vi "MDrive_Get_Variable.vi"(3 "error in":errorcluster, 4 "Variable":string, 5 "VISA resource name in":refnum<visa-resource-name>) -> (0 "error out":errorcluster, 1 "number":i32, 2 "VISA resource name out":refnum<visa-resource-name>)   [LabVIEW 2010]
panel:
  out "substring":string
  out "String":string="\r\n"
  out "return count":u32
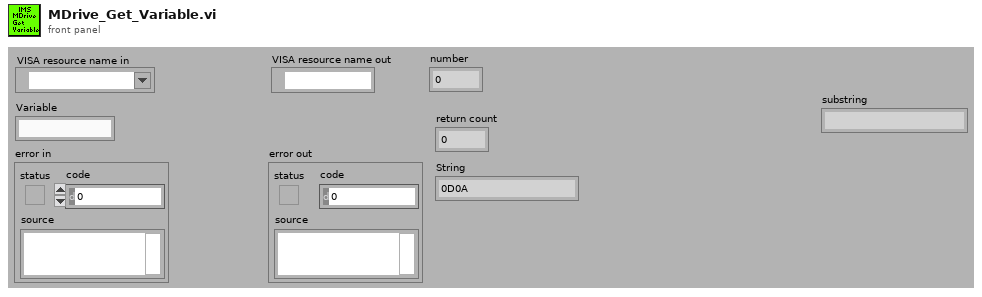
[diagram p1: front panel]
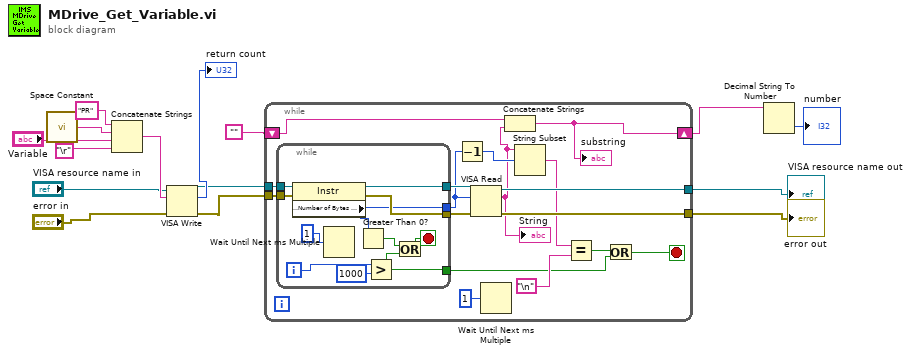
[diagram p0: block diagram]
diagram:
  n1 = call <vilib>:"Space Constant.vi"() -> ("String"=w12:string)
  n2 = Concatenate Strings("PR" ("string"), w12, "Variable", "\r") -> (w15:string)
  n3 = VISA Write(VISA resource name="VISA resource name in", write buffer=w15, error in (no error)="error in") -> (VISA resource name out=w6:refnum<visa-resource-name>, return count=→"return count":u32, error out=w5:errorcluster)
  n4 = while {
    tunnel: w6 -> [w30]
    tunnel: w5 -> [w29]
    tunnel: [w28] -> w3
    tunnel: [w27] -> w2
    shift-right: [w21] -> w1
    shift-left: "" -> [w22]
    stop <- w17 stop-if-true
    n5 = while {
      tunnel: [w43] -> w32
      tunnel: [w42] -> w31
      tunnel: w30 -> [w41]
      tunnel: w29 -> [w40]
      tunnel: [w39] -> w25
      tunnel: [w33] -> w18
      i -> [w37]
      stop <- w34 stop-if-true
      n6 = property class="Instr"(reference=w41, error in=w40) -> (reference out=w43:refnum<visa-resource-name>, error out=w42:errorcluster, "Serial Settings:Number of Bytes at Serial Port"=w39:u32)
      n7 = Wait Until Next ms Multiple(millisecond multiple=u32 1) -> ()  [unwired: 1 out]
      n8 = Greater Than 0?(x=w39) -> (x > 0?=w35:bool)
      n9 = Greater?(x=w37, y=1000) -> (0:w33:bool)
      n10 = Or(x=w35, y=w33) -> (x .or. y?=w34:bool)
    }
    n11 = Decrement(x=w25) -> (x-1=w24:u32)
    n12 = VISA Read(VISA resource name=w32, byte count=w25, error in (no error)=w31) -> (VISA resource name out=w28:refnum<visa-resource-name>, read buffer=w16:string, error out=w27:errorcluster)  [unwired: 1 out]
    "String" <- w16
    n13 = Wait Until Next ms Multiple(millisecond multiple=u32 1) -> ()  [unwired: 1 out]
    n14 = Concatenate Strings(w22, w16) -> (w21:string)
    "substring" <- w21
    n15 = String Subset(string=w16, offset (0)=w24) -> (substring=w23:string)  [unwired: 1 in]
    n16 = Equal?(x=w23, y="\n") -> (x = y?=w19:bool)
    n17 = Or(x=w19, y=w18) -> (x .or. y?=w17:bool)
  }
  "error out" <- w2
  "VISA resource name out" <- w3
  n18 = Decimal String To Number(string=w1) -> (number=→"number":i32)  [unwired: 2 in, 1 out]
